vi "Variance SubVI.vi"(0 "Calibration in":T1, 7 "Data in":dbl[][](array[numeric])) -> (1 "GyrX":T4, 2 "GyrY":T4, 3 "GyrZ":T4, 4 "Calibration out":T1, 8 "AccX":T4, 10 "AccY":T4, 12 "MagX":T4, 13 "MagY":T4, 14 "MagZ":T4, 15 "AccZ":T4)   [LabVIEW 2021, in "IMU Processing.lvlib"]
uses:
  IMU Processing.lvlib
  Calibration configuration.ctl
  Gyroscope calibration.ctl
  Accerelometer calibration.ctl
  <vilib>/Analysis/NI_AALBase.lvlib
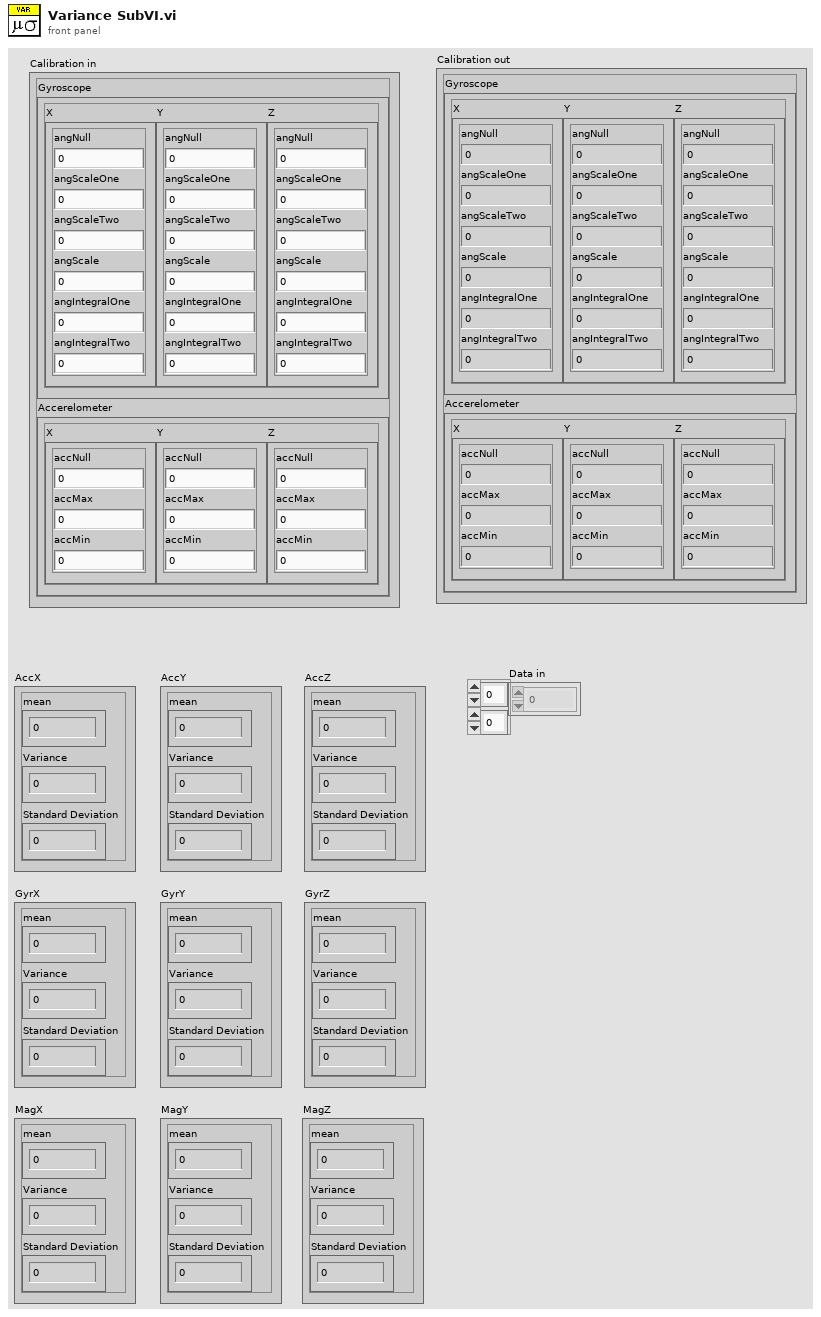
[diagram p1: front panel]
types:
  T1 = typedef "IMU Processing.lvlib/Calibration configuration.ctl" = cluster{"Gyroscope":cluster{"X":T2, "Y":T2, "Z":T2}, "Accerelometer":cluster{"X":T3, "Y":T3, "Z":T3}}
  T2 = typedef "IMU Processing.lvlib/Gyroscope calibration.ctl" = cluster{"angNull":dbl, "angScaleOne":dbl, "angScaleTwo":dbl, "angScale":dbl, "angIntegralOne":dbl, "angIntegralTwo":dbl}
  T3 = typedef "IMU Processing.lvlib/Accerelometer calibration.ctl" = cluster{"accNull":dbl, "accMax":dbl, "accMin":dbl}
  T4 = cluster{"mean":dbl, "Variance":dbl, "Standard Deviation":dbl}
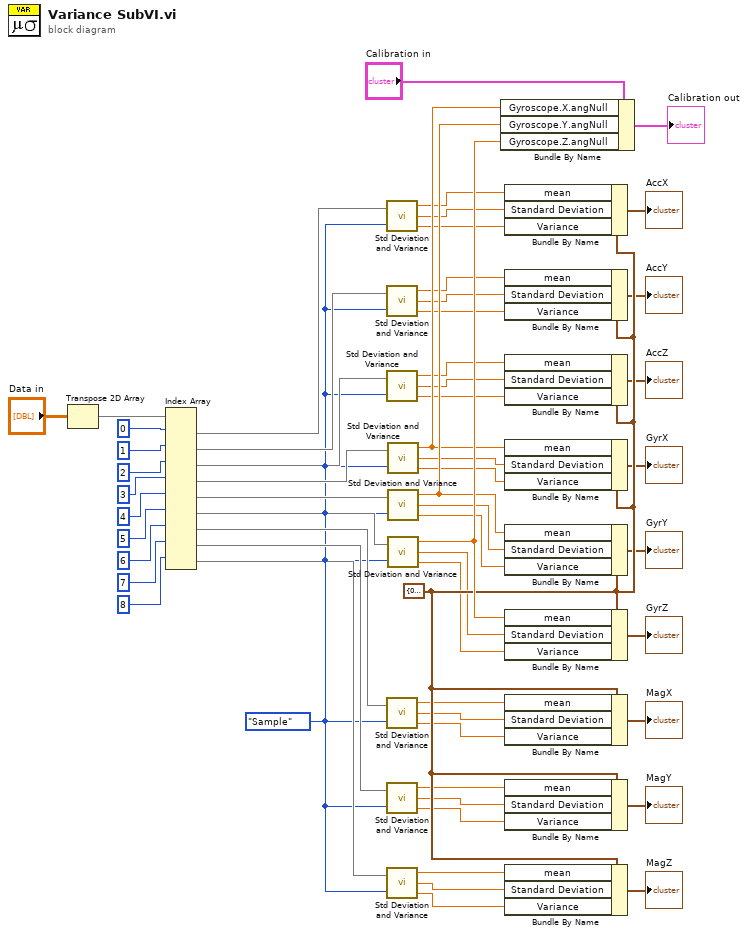
[diagram p0: block diagram]
diagram:
  w54 = T4 {"mean"=0.0, "Variance"=0.0, "Standard Deviation"=0.0} ("Statistics")
  w10 = enum16{"Sample", "Population"}."Sample" ("Weighting (Sample)")
  n1 = Transpose 2D Array(2D array="Data in") -> (transposed array=w1:dbl[][])
  n2 = Index Array(array=w1, index (row) #1=0 ("index (row)"), index (row) #2=1 ("index (row)"), index (row) #3=2 ("index (row)"), index (row) #4=3 ("index (row)"), index (row) #5=4 ("index (row)"), index (row) #6=5 ("index (row)"), index (row) #7=6 ("index (row)"), index (row) #8=7 ("index (row)"), index (row) #9=8 ("index (row)")) -> (element #1=w9:dbl[], element #2=w11:dbl[], element #3=w12:dbl[], element #4=w13:dbl[], element #5=w14:dbl[], element #6=w15:dbl[], element #7=w55:dbl[], element #8=w19:dbl[], element #9=w20:dbl[])  [unwired: 9 in]
  n3 = call <vilib>:"Std Deviation and Variance.vi"("X"=w9, "Weighting (Sample)"=w10) -> ("mean"=w21:dbl, "standard deviation"=w22:dbl, "variance"=w23:dbl)
  n4 = call <vilib>:"Std Deviation and Variance.vi"("X"=w11, "Weighting (Sample)"=w10) -> ("mean"=w26:dbl, "standard deviation"=w27:dbl, "variance"=w28:dbl)
  n5 = call <vilib>:"Std Deviation and Variance.vi"("X"=w12, "Weighting (Sample)"=w10) -> ("mean"=w29:dbl, "standard deviation"=w30:dbl, "variance"=w31:dbl)
  n6 = call <vilib>:"Std Deviation and Variance.vi"("X"=w55, "Weighting (Sample)"=w10) -> ("mean"=w38:dbl, "standard deviation"=w39:dbl, "variance"=w40:dbl)
  n7 = call <vilib>:"Std Deviation and Variance.vi"("X"=w19, "Weighting (Sample)"=w10) -> ("mean"=w41:dbl, "standard deviation"=w42:dbl, "variance"=w43:dbl)
  n8 = call <vilib>:"Std Deviation and Variance.vi"("X"=w20, "Weighting (Sample)"=w10) -> ("mean"=w44:dbl, "standard deviation"=w45:dbl, "variance"=w46:dbl)
  n9 = call <vilib>:"Std Deviation and Variance.vi"("X"=w13, "Weighting (Sample)"=w10) -> ("mean"=w58:dbl, "standard deviation"=w32:dbl, "variance"=w33:dbl)
  n10 = call <vilib>:"Std Deviation and Variance.vi"("X"=w14, "Weighting (Sample)"=w10) -> ("mean"=w59:dbl, "standard deviation"=w34:dbl, "variance"=w35:dbl)
  n11 = call <vilib>:"Std Deviation and Variance.vi"("X"=w15, "Weighting (Sample)"=w10) -> ("mean"=w60:dbl, "standard deviation"=w36:dbl, "variance"=w37:dbl)
  n12 = Bundle By Name(cluster="Calibration in", "Gyroscope.X.angNull"=w58, "Gyroscope.Y.angNull"=w59, "Gyroscope.Z.angNull"=w60) -> (→"Calibration out":T1)
  n13 = Bundle By Name(cluster=w54, "mean"=w21, "Standard Deviation"=w22, "Variance"=w23) -> (→"AccX":T4)
  n14 = Bundle By Name(cluster=w54, "mean"=w26, "Standard Deviation"=w27, "Variance"=w28) -> (→"AccY":T4)
  n15 = Bundle By Name(cluster=w54, "mean"=w29, "Standard Deviation"=w30, "Variance"=w31) -> (→"AccZ":T4)
  n16 = Bundle By Name(cluster=w54, "mean"=w58, "Standard Deviation"=w32, "Variance"=w33) -> (→"GyrX":T4)
  n17 = Bundle By Name(cluster=w54, "mean"=w59, "Standard Deviation"=w34, "Variance"=w35) -> (→"GyrY":T4)
  n18 = Bundle By Name(cluster=w54, "mean"=w60, "Standard Deviation"=w36, "Variance"=w37) -> (→"GyrZ":T4)
  n19 = Bundle By Name(cluster=w54, "mean"=w38, "Standard Deviation"=w39, "Variance"=w40) -> (→"MagX":T4)
  n20 = Bundle By Name(cluster=w54, "mean"=w41, "Standard Deviation"=w42, "Variance"=w43) -> (→"MagY":T4)
  n21 = Bundle By Name(cluster=w54, "mean"=w44, "Standard Deviation"=w45, "Variance"=w46) -> (→"MagZ":T4)
